vi "init wrapper.vi"(8 "error in (no error)":errorcluster, 10 "module configuration":refnum<class "TBM module configuration.lvclass">, 11 "module in":refnum<class "TBM module execution interface.lvclass">) -> (0 "error out":errorcluster, 1 "data allocations":T1, 2 "execution settings":T4, 3 "module out":refnum<class "TBM module execution interface.lvclass">)   [LabVIEW 2013, in "TBM module execution interface.lvclass"]
uses:
  TBM module execution interface.lvclass
  execution settings.ctl
  channel/data tables.ctl
  <vilib>/NI/Tag Bus/dictionary/data dictionary.lvclass
  <vilib>/NI/Tag Bus/dictionary table pair.ctl
  <vilib>/NI/Tag Bus/table/data table.ctl
  module configuration/TBM module configuration.lvclass
  <vilib>/NI/Syslog Wrapper - Linux/write syslog.vi
  <vilib>/Utility/LVClass/Get LV Class Name.vi
  <vilib>/NI/Tag Bus/table/data table.lvlib
  <vilib>/NI/Tag Bus/tag bus.lvlib
  channel/TBM channel.lvclass
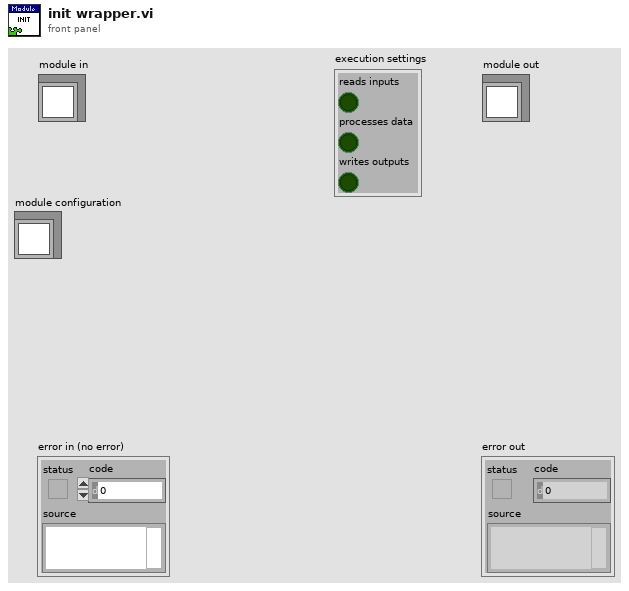
[diagram p1: front panel]
types:
  T1 = typedef "TBM channel.lvclass/data tables.ctl" = cluster{"input data":T2, "processing parameter":T2, "processing result":T2, "output data":T2}
  T2 = typedef "tag bus.lvlib/dictionary table pair.ctl" = cluster{"data dictionary":refnum<class "data dictionary.lvclass">, "data table":T3}
  T3 = typedef "tag bus.lvlib/data table.lvlib/data table.ctl" = cluster{"Double":dbl[], "Single":sgl[], "I64":i64[], "I32":i32[], "I16":i16[], "I8":i8[], "U64":u64[], "U32":u32[], "U16":u16[], "U8":u8[], "Boolean":bool[], "String":string[], "Array of Double":cluster{"DBL Array":dbl[]}[], "Array of Single":cluster{"SGL Array":sgl[]}[], "Array of I64":cluster{"I64 Array":i64[]}[], "Array of I32":cluster{"I32 Array":i32[]}[], "Array of I16":cluster{"I16 Array":i16[]}[], "Array of I8":cluster{"I8 Array":i8[]}[], "Array of U64":cluster{"U64 Array":u64[]}[], "Array of U32":cluster{"U32 Array":u32[]}[], "Array of U16":cluster{"U16 Array":u16[]}[], "Array of U8":cluster{"U8 Array":u8[]}[], "Array of Boolean":cluster{"Boolean Array":bool[]}[], "Array of String":cluster{"String Array":string[]}[]}
  T4 = typedef "TBM module execution interface.lvclass/execution settings.ctl" = cluster{"reads inputs":bool, "processes data":bool, "writes outputs":bool}
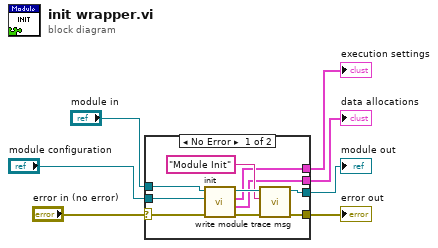
[diagram p0: block diagram]
diagram:
  n1 = case shown="No Error" "error in (no error)" {
    selector: "error in (no error)" -> [w16 w19]
    tunnel: [w12 w19] -> w6
    tunnel: [w11 w18] -> w4
    tunnel: "module in" -> [w17 w18]
    tunnel: [w10 _] -> w3
    tunnel: [w9 _] -> w2
    tunnel: "module configuration" -> [w8 _]
    frame No Error {
      n2 = call-dynamic "init.vi"("error in"=w16, "module configuration"=w8, "module in"=w17) -> ("error out"=w14:errorcluster, "data allocations"=w9:T1, "execution settings"=w10:T4, "module out"=w15:refnum<class "TBM module execution interface.lvclass">)  [unwired: 5 in]
      n3 = call "write module trace msg.vi"("error in (no error)"=w14, "message"="Module Init", "module in"=w15) -> ("error out"=w12:errorcluster, "module out"=w11:refnum<class "TBM module execution interface.lvclass">)  [unwired: 7 in]
    }
    frame Error {
    }
  }
  "error out" <- w6
  "module out" <- w4
  "execution settings" <- w3
  "data allocations" <- w2
